vi "LauncherFA.vi"() -> ()   [LabVIEW 2020]
uses:
  FirstActor.lvclass
  C:/Program Files (x86)/National Instruments/LabVIEW 2020/vi.lib/ActorFramework/Actor/Actor.lvclass
  <vilib>/ActorFramework/Message Enqueuer/Message Enqueuer.lvclass/Message Enqueuer.ctl
  <vilib>/ActorFramework/Message Enqueuer/Enqueue.vi
  FirstActor Messages/Saludo Msg/Saludo Msg.lvclass
  C:/Program Files (x86)/National Instruments/LabVIEW 2020/vi.lib/ActorFramework/Message/Message.lvclass
  <vilib>/ActorFramework/Stop Msg/Stop Msg.lvclass
  <vilib>/ActorFramework/Message Priority Queue/Priority Enqueue.vi
  <vilib>/ActorFramework/Actor/Actor.lvclass
panel:
  in  "Mensaje":bool
  in  "stop":bool
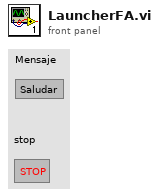
[diagram p1: front panel]
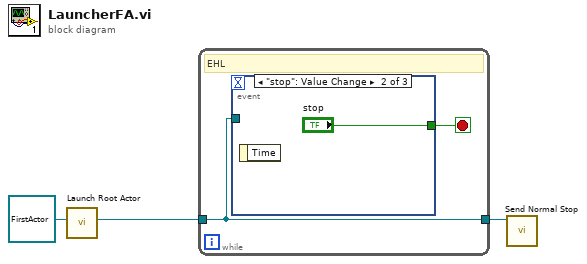
[diagram p0: block diagram]
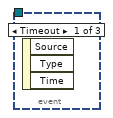
[diagram p2: hidden frame]
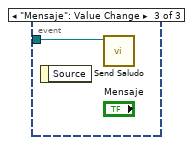
[diagram p3: hidden frame]
diagram:
  n1 = call <vilib>:"Launch Root Actor.vi"("Actor"=refnum<class "FirstActor.lvclass"> refnum ("FirstActor.lvlib:FirstActor.lvclass")) -> ("Actor's Enqueuer"=w3:refnum<class "Message Enqueuer.lvclass">)  [unwired: 9 in, 1 out]
  n2 = while {
    tunnel: w3 -> [w4]
    tunnel: [w4] -> w2
    stop <- w5 stop-if-true
    # "EHL"
    n3 = event shown="[1] \"stop\": Value Change" {
      selector: _ -> [_ _ _]
      dyn-events: _ -> [_ _ _]
      timeout: _ -> [_ _ _]
      tunnel: [_ "stop" _] -> w5
      tunnel: w4 -> [_ _ w7]
      event Timeout {
        n4 = event-data() -> ()  [unwired: 1 in, 3 out]
      }
      event "stop": Value Change {
        n5 = event-data() -> ()  [unwired: 1 in, 1 out]
      }
      event "Mensaje": Value Change {
        n6 = event-data() -> ()  [unwired: 1 in, 1 out]
        n7 = call "Send Saludo.vi"("Message Enqueuer"=w7) -> ()  [unwired: 9 in, 2 out]
      }
    }
  }
  n8 = call <vilib>:"Send Normal Stop.vi"("Message Enqueuer"=w2) -> ()  [unwired: 10 in, 1 out]
